vi "Cull and Group Vertical.vi"(9 "Score Cutoff":dbl=50.0, 10 "Sorted Data":dbl[][](array[numeric])) -> (0 "Rect":T1, 1 "Top Score":dbl, 3 "Center":cluster{"X":dbl, "Y":dbl})   [LabVIEW 2025]
doc: "Examine the particle measurements to find the most likely pair that make up the target. This mostly compares the edges of the bounding boxes. It then returns information about the overall target, notably the rectangle sourrounding the particles, the vertical line that bisects the target, and the center of the top particle."
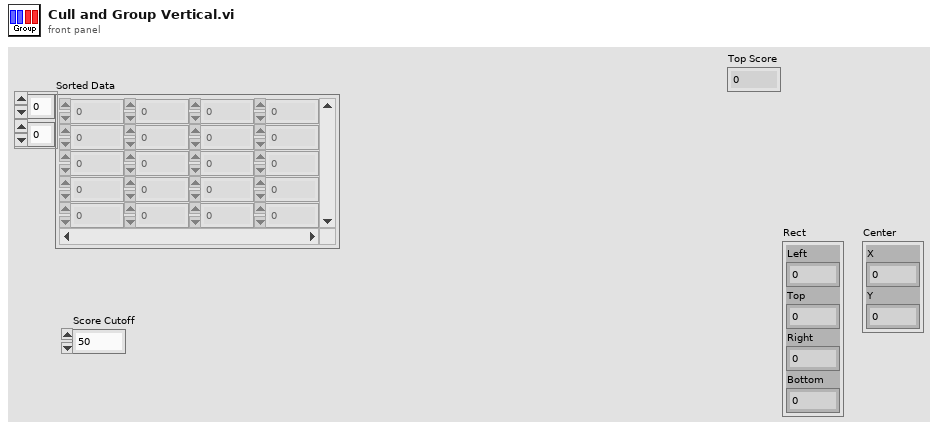
[diagram p1: front panel]
types:
  T1 = cluster{"Left":dbl, "Top":dbl, "Right":dbl, "Bottom":dbl}
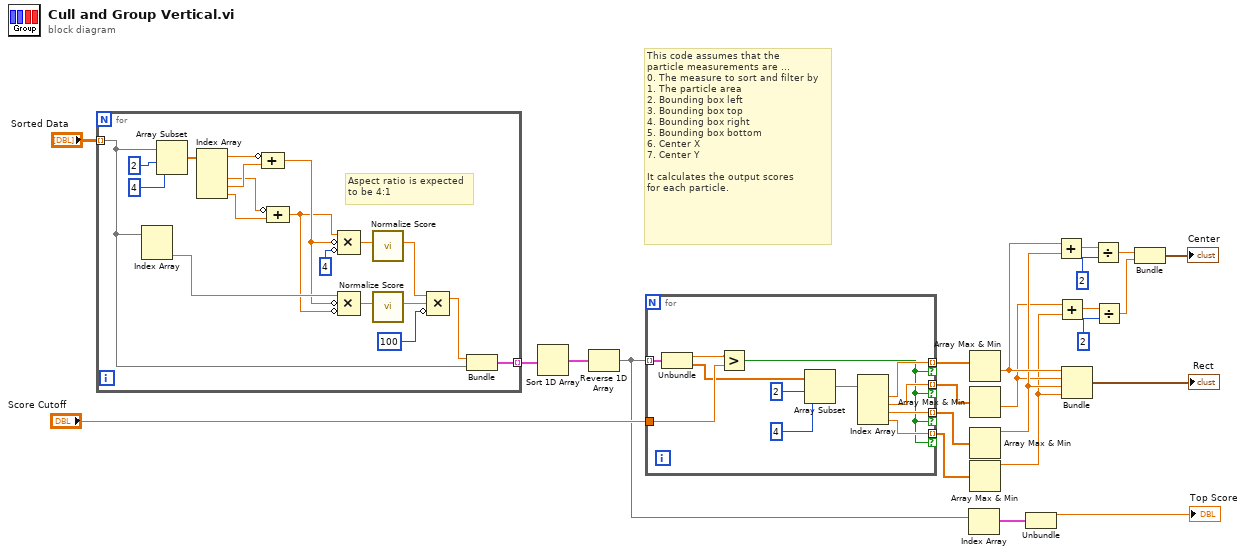
[diagram p0: block diagram]
diagram:
  # "This code assumes that the\nparticle measurements are ...\n0. The measure to sort and filter by\n1. The particle area\n2. Bounding box left\n3. Bounding box top\n4. Bounding box right\n5. Bounding box bottom\n6. Center X\n7. Center Y\n\nIt calculates the output scores\nfor each particle."
  n1 = for {
    tunnel: "Sorted Data" -> [w26] mode=indexing
    tunnel: [w24] -> w22 mode=indexing
    # "Aspect ratio is expected\nto be 4:1"
    n2 = Index Array(array=w26) -> (element #2=w33:dbl)  [unwired: 2 in, 1 out]
    n3 = Array Subset(array=w26, index=2, length=4) -> (w40:dbl[])
    n4 = Index Array(array=w40) -> (element #1=w38:dbl, element #2=w36:dbl, element #3=w39:dbl, element #4=w37:dbl)  [unwired: 4 in]
    n5 = Compound Arithmetic op=ADD(invert w38, w39) -> (w32:dbl)
    n6 = Compound Arithmetic op=ADD(invert w36, w37) -> (w31:dbl)
    n7 = Compound Arithmetic op=MULTIPLY(w31, invert w32, invert 4 ("length")) -> (w34:dbl)
    n8 = Compound Arithmetic op=MULTIPLY(w33, invert w32, invert w31) -> (w30:dbl)
    n9 = call "Normalize Score.vi"("Value"=w34) -> ("Score"=w29:dbl)  [unwired: 10 in]
    n10 = call "Normalize Score.vi"("Value"=w30) -> ("Score"=w28:dbl)  [unwired: 10 in]
    n11 = Compound Arithmetic op=MULTIPLY(w29, w28, invert 100 ("length")) -> (w25:dbl)
    n12 = Bundle(w25, "Sorted Data"=w26) -> (w24:cluster{dbl, "Sorted Data":dbl[]})  [unwired: 1 in]
  }
  n13 = Sort 1D Array(array=w22) -> (sorted array=w15:cluster{dbl, "Sorted Data":dbl[]}[])
  n14 = Reverse 1D Array(array=w15) -> (reversed array=w12:cluster{dbl, "Sorted Data":dbl[]}[])
  n15 = for {
    tunnel: w12 -> [w54] mode=indexing
    tunnel: "Score Cutoff" -> [w52]
    tunnel: [w47] -> w20 mode=indexing if=w43
    tunnel: [w46] -> w19 mode=indexing if=w43
    tunnel: [w45] -> w18 mode=indexing if=w43
    tunnel: [w44] -> w17 mode=indexing if=w43
    n16 = Unbundle(w54) -> (w53:dbl, "Sorted Data"=w48:dbl[])
    n17 = Greater?(x=w53, y=w52) -> (0:w43:bool)
    n18 = Array Subset(array=w48, index=2, length=4) -> (w51:dbl[])
    n19 = Index Array(array=w51) -> (element #1=w47:dbl, element #2=w46:dbl, element #3=w45:dbl, element #4=w44:dbl)  [unwired: 4 in]
  }
  n20 = Index Array(array=w12) -> (element=w14:cluster{dbl, "Sorted Data":dbl[]})  [unwired: 1 in]
  n21 = Array Max & Min(array=w20) -> (min value=w9:dbl)  [unwired: 3 out]
  n22 = Array Max & Min(array=w19) -> (min value=w5:dbl)  [unwired: 3 out]
  n23 = Array Max & Min(array=w18) -> (max value=w8:dbl)  [unwired: 3 out]
  n24 = Array Max & Min(array=w17) -> (max value=w4:dbl)  [unwired: 3 out]
  n25 = Unbundle(w14) -> (→"Top Score":dbl)  [unwired: 1 out]
  n26 = Add(x=w9, y=w8) -> (x+y=w10:dbl)
  n27 = Add(x=w5, y=w4) -> (x+y=w7:dbl)
  n28 = Bundle(w9, w5, w8, w4) -> (→"Rect":cluster{dbl, dbl, dbl, dbl})  [unwired: 1 in]
  n29 = Divide(x=w10, y=2 ("index")) -> (x/y=w3:dbl)
  n30 = Divide(x=w7, y=2 ("index")) -> (x/y=w2:dbl)
  n31 = Bundle(w3, w2) -> (→"Center":cluster{dbl, dbl})  [unwired: 1 in]
